vi "csuCloseShutter.vi"() -> ()   [LabVIEW 2017]
doc: "SubVI for sending commands to the MAC5000 and receiving responses from the MAC5000."
uses:
  globalDevices.vi
panel:
  out "Raw Response":string
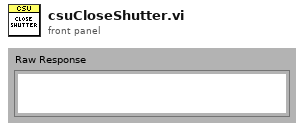
[diagram p1: front panel]
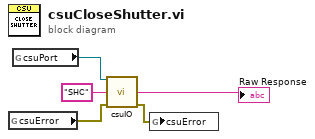
[diagram p0: block diagram]
diagram:
  n1 = global read "globalDevices.vi" "csuError"() -> (w2:errorcluster)
  n2 = global read "globalDevices.vi" "csuPort"() -> (w3:refnum<visa-resource-name>)
  n3 = call "csuIO.vi"("VISA  IN"=w3, "Command (to ctlr)"="SHC", "error in"=w2) -> ("Raw Response"=→"Raw Response":string, "error out"=w1:errorcluster)  [unwired: 9 in, 2 out]
  n4 = global write "globalDevices.vi" "csuError"(w1) -> ()
